vi "HiReWFS initialize.vi"(11 "error in (no error)":errorcluster) -> (2 "IsConnected 2":bool, 3 "Open":refnum<k24>, 4 ".NET Refnum out":refnum<k24>, 6 "IsOpen 2":bool, 8 "Parameters":refnum<k24>, 10 "IsConnected":bool, 13 "IsOpen":bool, 14 "StreamGrabber":refnum<k24>, 15 "error out":errorcluster)   [LabVIEW 2023, in "HiResWFS.lvclass"]
uses:
  HiResWFS.lvclass
  Basler.Pylon
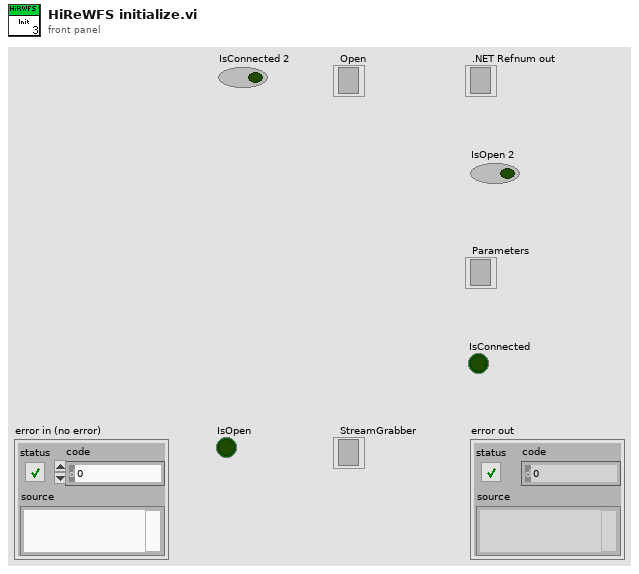
[diagram p1: front panel]
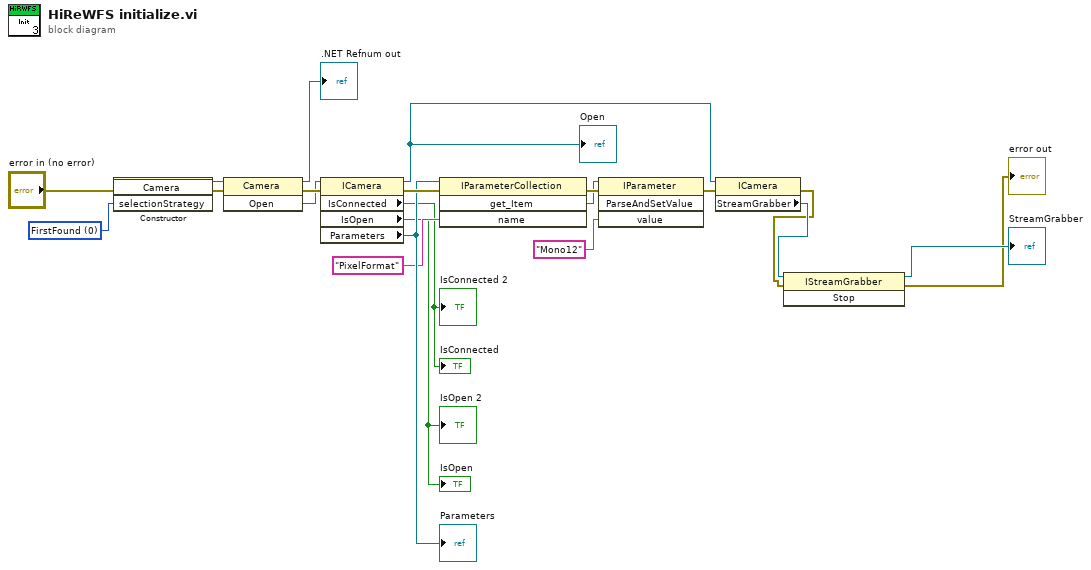
[diagram p0: block diagram]
diagram:
  w7 = 0 items=["FirstFound", "Unambiguous"] ("selectionStrategy")
  n1 = constructor class="Camera"(error in="error in (no error)", "selectionStrategy"=w7) -> (reference out=w8:refnum<k24>, error out=w6:errorcluster)  [unwired: 2 in, 2 out]
  n2 = invoke class="Camera" method="Open"(reference=w8, error in=w6) -> (reference out=→".NET Refnum out":refnum<k24>, error out=w12:errorcluster, "Open"=w5:refnum<k24>)  [unwired: 1 in]
  n3 = property class="ICamera"(reference=w5, error in=w12) -> (reference out=w14:refnum<k24>, error out=w19:errorcluster, "IsConnected"=→"IsConnected" →"IsConnected 2":bool, "IsOpen"=→"IsOpen" →"IsOpen 2":bool, "Parameters"=w18:refnum<k24>)
  "Parameters" <- w18
  "Open" <- w14
  n4 = invoke class="IParameterCollection" method="get_Item"(reference=w18, error in=w19, "name"="PixelFormat") -> (error out=w20:errorcluster, "get_Item"=w17:refnum<k24>)  [unwired: 1 in, 2 out]
  n5 = invoke class="IParameter" method="ParseAndSetValue"(reference=w17, error in=w20, "value"="Mono12" ("name")) -> (error out=w21:errorcluster)  [unwired: 1 in, 3 out]
  n6 = property class="ICamera"(reference=w14, error in=w21) -> (error out=w2:errorcluster, "StreamGrabber"=w4:refnum<k24>)  [unwired: 1 out]
  n7 = invoke class="IStreamGrabber" method="Stop"(reference=w4, error in=w2) -> (reference out=→"StreamGrabber":refnum<k24>, error out=→"error out":errorcluster)  [unwired: 1 in, 1 out]
